vi "Ask to Close App.vi"(8 "error in":errorcluster) -> (0 "error out":errorcluster, 3 "T button?":bool)   [LabVIEW 2024, in "User Interface.lvlib"]
uses:
  User Interface.lvlib
  UI Queue - Enqueue.vi
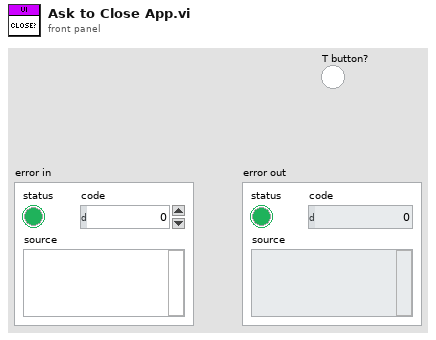
[diagram p1: front panel]
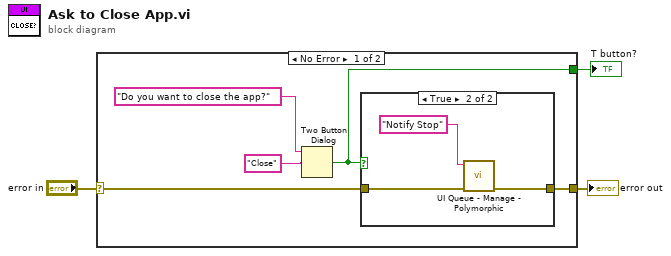
[diagram p0: block diagram]
diagram:
  n1 = case shown="No Error" "error in" {
    selector: "error in" -> [w6 w13]
    tunnel: [w5 w13] -> w3
    tunnel: [w4 _] -> w1
    frame No Error {
      n2 = Two Button Dialog(message="Do you want to close the app?", 2:"Close" ("T button name (\"OK\")")) -> (T button?=w4:bool)  [unwired: 1 in]
      n3 = case shown="True" w4 {
        tunnel: w6 -> [w9 w12]
        tunnel: [w9 w11] -> w5
        frame False {
        }
        frame True {
          n4 = call-poly "UI Queue - Manage - Polymorphic.vi"("error in"=w12, "Message"="Notify Stop") -> ("error out"=w11:errorcluster)  [unwired: 9 in]
        }
      }
    }
    frame Error {
    }
  }
  "error out" <- w3
  "T button?" <- w1
